vi "engine.poststep.next-handler.vi"(8 "error in":errorcluster, 9 "NEXT/PREV":enum16{"NEXT", "PREV"}(ring), 11 "Proc Element in":variant) -> (0 "error out":errorcluster, 3 "Proc Element out":variant)   [LabVIEW 2024]
uses:
  controls/typeProcVarientName.ctl
  Polymorphics/variantCtrlNumber.vi
  proc.util.validateParamExist.vi
  <vilib>/Utility/error.llb/Clear Errors.vi
  util.error.create.vi
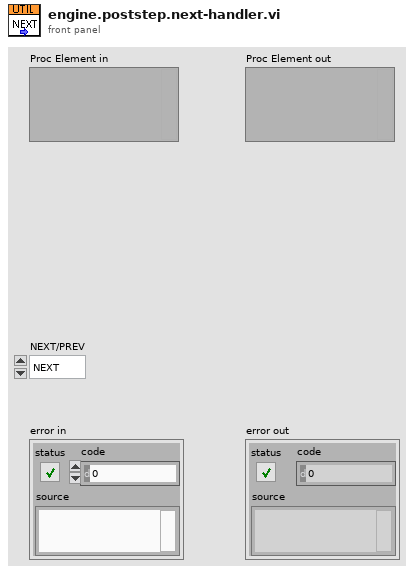
[diagram p1: front panel]
types:
  T1 = typedef "typeProcVarientName.ctl" = enum16{"procNameID", "procModuleID", "procPath", "procIsRunning", "procIndex", "procModule", "procRegisterNumeric", "procRegisterString", "procReport", "procReportPrev", "procCLK", "procStepPointer", "procType"}
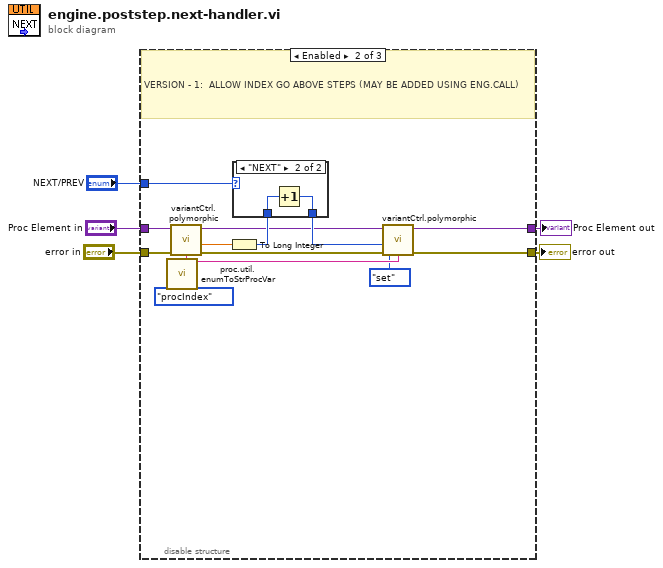
[diagram p0: block diagram]
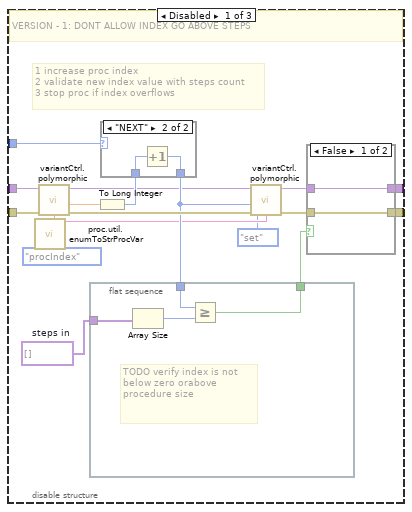
[diagram p2: hidden frame]
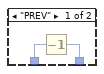
[diagram p3: hidden frame]
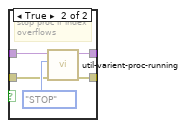
[diagram p4: hidden frame]
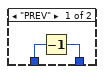
[diagram p5: hidden frame]
diagram:
  n1 = disable-structure shown="Enabled" {
    disable-tunnel: [w20 w49 _] -> w5
    disable-tunnel: [w19 w48 _] -> w4
    disable-tunnel: "Proc Element in" -> [w10 w40 _]
    disable-tunnel: "error in" -> [w9 w39 _]
    disable-tunnel: "NEXT/PREV" -> [w7 w37 _]
    frame Disabled {
      w6 = variant[] []  # steps in
      # "1 increase proc index\n2 validate new index value with steps count\n3 stop proc if index overflows"
      # "VERSION - 1: DONT ALLOW INDEX GO ABOVE STEPS"
      n2 = call "proc.util.enumToStrProcVar.vi"("Proc var"=typeProcVarientName."procIndex" ("name")) -> ("String"=w15:string)  [unwired: 10 in]
      n3 = call-poly "variantCtrl.polymorphic.vi"("error in"=w9, "name in"=w15, "variant in"=w10) -> ("error out"=w18:errorcluster, "number"=w12:dbl, "variant out"=w13:variant)  [unwired: 5 in, 1 out]
      n4 = flat-sequence {
        tunnel: [w26] -> w22
        tunnel: w16 -> [w25]
        tunnel: w6 -> [w24]
        frame #0 {
          # "TODO verify index is not below zero orabove procedure size"
          n5 = Array Size(array=w24) -> (size(s)=w23:i32)
          n6 = Greater Or Equal?(x=w25, y=w23) -> (x >= y?=w26:bool)
        }
      }
      n7 = To Long Integer(number=w12) -> (32bit integer=w17:i32)
      n8 = case shown="\"NEXT\"" w7 {
        tunnel: w17 -> [w28 w30]
        tunnel: [w27 w29] -> w16
        frame "PREV" {
          n9 = Decrement(x=w28) -> (x-1=w27:i32)
        }
        frame "NEXT" {
          n10 = Increment(x=w30) -> (x+1=w29:i32)
        }
      }
      n11 = call-poly "variantCtrl.polymorphic.vi"("menu in (get)"=enum16{"get", "set"}."set", "error in"=w18, "number"=w16, "name in"=w15, "variant in"=w13) -> ("error out"=w21:errorcluster, "variant out"=w14:variant)  [unwired: 3 in, 2 out]
      n12 = case shown="False" w22 {
        tunnel: w14 -> [w32 w36]
        tunnel: [w32 w34] -> w19
        tunnel: [w31 w33] -> w20
        tunnel: w21 -> [w31 w33]
        frame False {
        }
        frame True {
          # "stop proc if index overflows"
          n13 = call "util-varient-proc-running.vi"("Enum"=enum16{"START", "STOP"}."STOP", "Procedure in"=w36) -> ("Procedure out"=w34:variant)  [unwired: 8 in, 1 out]
        }
      }
    }
    frame Enabled {
      # "VERSION - 1:  ALLOW INDEX GO ABOVE STEPS (MAY BE ADDED USING ENG.CALL)"
      n14 = call "proc.util.enumToStrProcVar.vi"("Proc var"=typeProcVarientName."procIndex" ("name")) -> ("String"=w44:string)  [unwired: 10 in]
      n15 = call-poly "variantCtrl.polymorphic.vi"("error in"=w39, "name in"=w44, "variant in"=w40) -> ("error out"=w47:errorcluster, "number"=w42:dbl, "variant out"=w43:variant)  [unwired: 5 in, 1 out]
      n16 = To Long Integer(number=w42) -> (32bit integer=w46:i32)
      n17 = case shown="\"NEXT\"" w37 {
        tunnel: w46 -> [w51 w53]
        tunnel: [w50 w52] -> w45
        frame "PREV" {
          n18 = Decrement(x=w51) -> (x-1=w50:i32)
        }
        frame "NEXT" {
          n19 = Increment(x=w53) -> (x+1=w52:i32)
        }
      }
      n20 = call-poly "variantCtrl.polymorphic.vi"("menu in (get)"=enum16{"get", "set"}."set", "error in"=w47, "number"=w45, "name in"=w44, "variant in"=w43) -> ("error out"=w49:errorcluster, "variant out"=w48:variant)  [unwired: 3 in, 2 out]
    }
    frame Disabled {
    }
  }
  "error out" <- w5
  "Proc Element out" <- w4
